vi "getKickForceFromDistance.vi"(4 "multiplicativeFactorToPassForce":dbl, 6 "multiplicativeFactorToKickForce":dbl, 8 "error in (no error)":errorcluster, 9 "pass?":bool=TRUE, 10 "distance":dbl format="%#_13g", 11 "Game in":refnum<class "Game.lvclass">) -> (0 "error out":errorcluster, 2 "kickForce":dbl, 3 "Game out":refnum<class "Game.lvclass">)   [LabVIEW 2020, in "Game.lvclass"]
uses:
  Game.lvclass
panel:
  in  "PassForceMean(default)":dbl[][](array[numeric])=[[7290.431216910258, 40.0, 0.0], [5588.112993733975, 38.0, 1.0], [3875.3759268249646, 36.0, 2.0], [2774.3232323929033, 34.0, 3.0], [1734.3636422844513, 32.0, 4.0], [1245.8077164192352, 30.0, 5.0], [999.2424946413078, 28.0, 6.0], [814.8573524752643, 26.0, 7.0], [0.0, 24.0, -1.0]]
  in  "KickForceMean(default)":dbl[][](array[numeric])=[[4656.29801400436, 70.0, 0.0], [4335.279054852332, 65.0, 1.0], [3230.618228702577, 60.0, 2.0], [2278.855764894509, 55.0, 3.0], [1340.6494904493466, 50.0, 4.0], [0.0, 45.0, -1.0]]
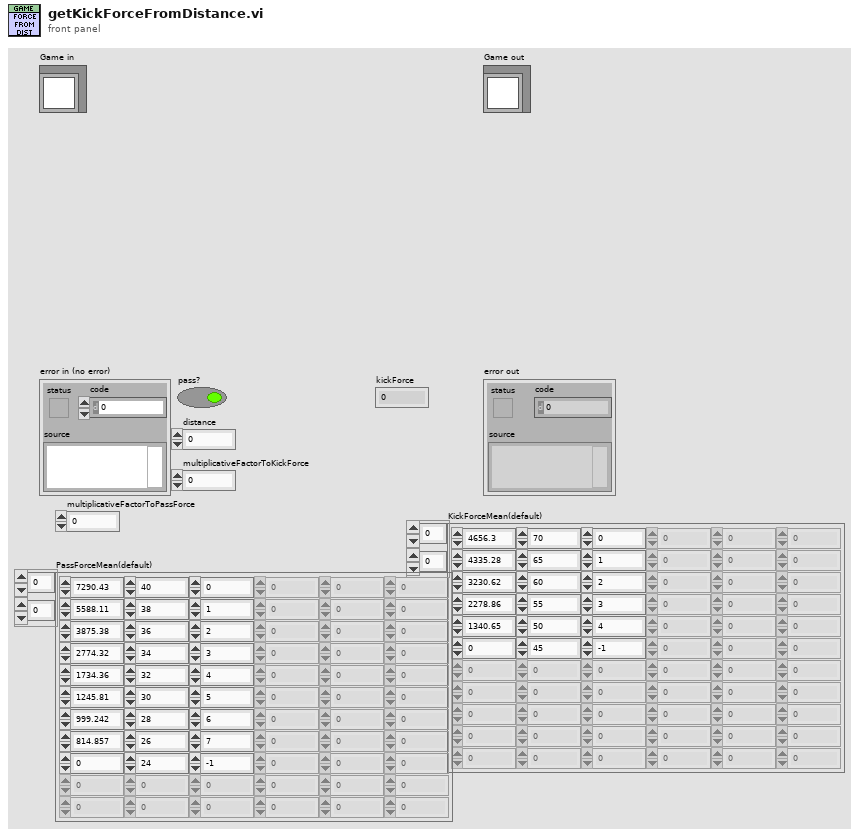
[diagram p1: front panel]
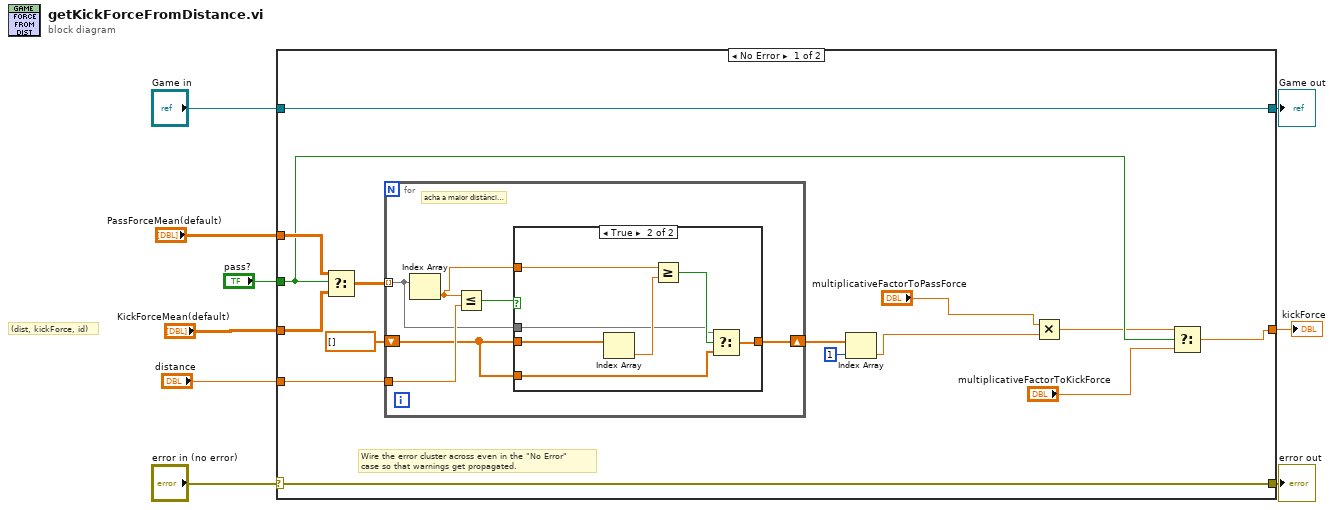
[diagram p0: block diagram]
diagram:
  # "(dist, kickForce, id)"
  n1 = case shown="No Error" "error in (no error)" {
    selector: "error in (no error)" -> [w23 w40]
    tunnel: [w23 w40] -> w8
    tunnel: [w24 w39] -> w6
    tunnel: "Game in" -> [w24 w39]
    tunnel: "pass?" -> [w13 _]
    tunnel: "PassForceMean(default)" -> [w22 _]
    tunnel: "KickForceMean(default)" -> [w21 _]
    tunnel: "distance" -> [w19 _]
    tunnel: [w10 _] -> w1
    frame No Error {
      # "Wire the error cluster across even in the \"No Error\"\ncase so that warnings get propagated."
      n2 = Select(t=w22, s=w13, f=w21) -> (s? t:f=w20:dbl[][])
      n3 = for {
        tunnel: w20 -> [w27] mode=indexing
        tunnel: w19 -> [w30]
        shift-right: [w25] -> w17
        shift-left: dbl[] [] ("KickForceMean(default)") -> [w26]
        # "acha a maior distância menor ou igual à distancia que vou chutar"
        n4 = Index Array(array=w27) -> (element=w28:dbl)  [unwired: 1 in]
        n5 = Less Or Equal?(x=w28, y=w30) -> (x <= y?=w29:bool)
        n6 = case shown="True" w29 {
          tunnel: w26 -> [w31 w38]
          tunnel: w28 -> [_ w37]
          tunnel: w27 -> [_ w34]
          tunnel: w26 -> [_ w33]
          tunnel: [w31 w32] -> w25
          frame False {
          }
          frame True {
            n7 = Index Array(array=w38) -> (element=w36:dbl)  [unwired: 1 in]
            n8 = Greater Or Equal?(x=w37, y=w36) -> (x >= y?=w35:bool)
            n9 = Select(t=w34, s=w35, f=w33) -> (s? t:f=w32:dbl[])
          }
        }
      }
      n10 = Index Array(array=w17, index=1) -> (element=w15:dbl)
      n11 = Multiply(x="multiplicativeFactorToPassForce", y=w15) -> (x*y=w12:dbl)
      n12 = Select(t=w12, s=w13, f="multiplicativeFactorToKickForce") -> (s? t:f=w10:dbl)
    }
    frame Error {
    }
  }
  "error out" <- w8
  "Game out" <- w6
  "kickForce" <- w1
